vi "enumerateStaticDependencies.vi"(8 "error in (no error)":errorcluster, 11 "SMO.SelfTerminatingOverride":refnum<class "SMO.SelfTerminatingOverride.lvclass">) -> (0 "error out":errorcluster, 2 "Static Dependencies":refnum<class "Dependency.lvclass">[](array[class]), 3 "SMO.SelfTerminatingOverride out":refnum<class "SMO.SelfTerminatingOverride.lvclass">)   [LabVIEW 2021, in "SMO.SelfTerminatingOverride.lvclass"]
uses:
  SMO.SelfTerminatingOverride.lvclass
  SMO.SelfTerminatingOverride.lvclass/SMO.SelfTerminatingOverride.ctl
  SMO.SelfTerminating/SMO.SelfTerminating.lvclass
  src/Dependency/Dependency.lvclass
  src/SMO/SMO.lvclass
panel:
  # "For instructions on how to use the JKI State Machine Objects, examples and video tutorials, visit:\nhttp://jki.net/state-machine-objects/\n\nJKI State Machine Objects™\nhttp://jki.net/state-machine-objects/\nCopyright (C) 2005-2015, JKI <info@jki.net>\nALL RIGHTS RESERVED"
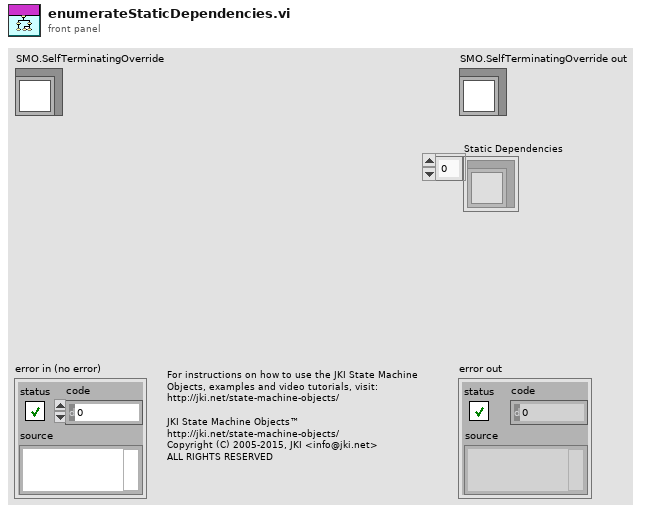
[diagram p1: front panel]
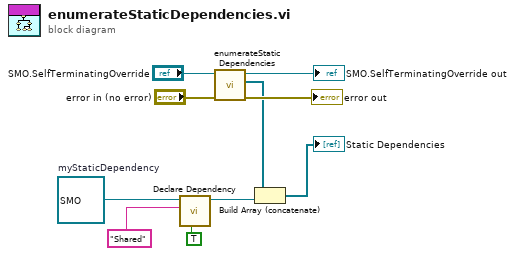
[diagram p0: block diagram]
diagram:
  w1 = refnum<class "SMO.lvclass"> refnum  # myStaticDependency
  n1 = call "Declare Dependency.vi"("Shared Resource (F)"=TRUE, "Name"="Shared", "Type"=w1) -> ("Dependency out"=w4:refnum<class "Dependency.lvclass">)  [unwired: 7 in, 1 out]
  n2 = call-parent "enumerateStaticDependencies.vi"("error in (no error)"="error in (no error)", "SMO"="SMO.SelfTerminatingOverride") -> ("error out"=→"error out":errorcluster, "Static Dependencies"=w6:refnum<class "Dependency.lvclass">[], "SMO out"=→"SMO.SelfTerminatingOverride out":refnum<class "SMO.SelfTerminatingOverride.lvclass">)  [unwired: 7 in]
  n3 = Build Array (concatenate)(w6, w4) -> (→"Static Dependencies":refnum<class "Dependency.lvclass">[])
